vi "Initialize Session.vi"(8 "error in (no error)":errorcluster, 11 "Python Toolkit in":refnum<class "Python Toolkit.lvclass">) -> (0 "error out":errorcluster, 3 "Python Toolkit out":refnum<class "Python Toolkit.lvclass">)   [LabVIEW 2018, in "Python Toolkit.lvclass"]
doc: "Initialize python session"
uses:
  Python Toolkit.lvclass
  Python Toolkit.lvclass/Python Toolkit.ctl
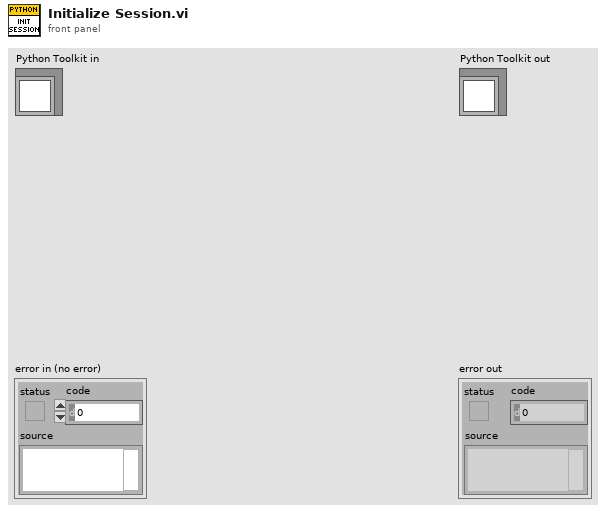
[diagram p1: front panel]
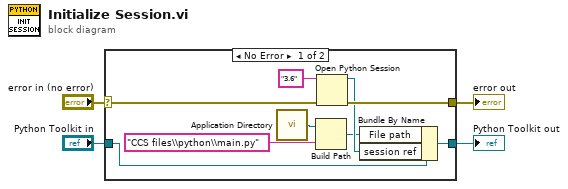
[diagram p0: block diagram]
diagram:
  n1 = case shown="No Error" "error in (no error)" {
    selector: "error in (no error)" -> [w10 w15]
    tunnel: [w9 w15] -> w3
    tunnel: [w12 w14] -> w1
    tunnel: "Python Toolkit in" -> [w13 w14]
    frame No Error {
      n2 = call <vilib>:"Application Directory.vi"() -> ("Application Directory"=w6:path)
      n3 = Build Path(base path=w6, name or relative path="CCS files\\python\\main.py") -> (appended path=w7:path)
      n4 = Open Python Session(python version="3.6" ("Python version"), 3:w10) -> (session out=w8:refnum<k35>, error out=w9:errorcluster)  [unwired: 1 in]
      n5 = Bundle By Name(cluster=w13, "File path"=w7, "session ref"=w8) -> (w12:refnum<class "Python Toolkit.lvclass">)
    }
    frame Error {
    }
  }
  "error out" <- w3
  "Python Toolkit out" <- w1
